vi "649Loops.vi"() -> ()   [LabVIEW 2023]
uses:
  <vilib>/numeric/Random Number (Range) U64.vi
  <vilib>/numeric/sub_Random U32.vi
  <vilib>/Utility/file.llb/Write Delimited Spreadsheet (string).vi
panel:
  in  "Append to file?":bool
  in  "file path (dialog if empty)":path
  out "?":u64[](array[numeric])
  out "?":u64[][](array[numeric])
  in  "?":bool
  # "6@49"
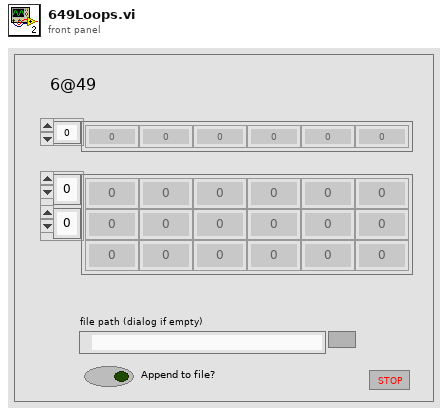
[diagram p1: front panel]
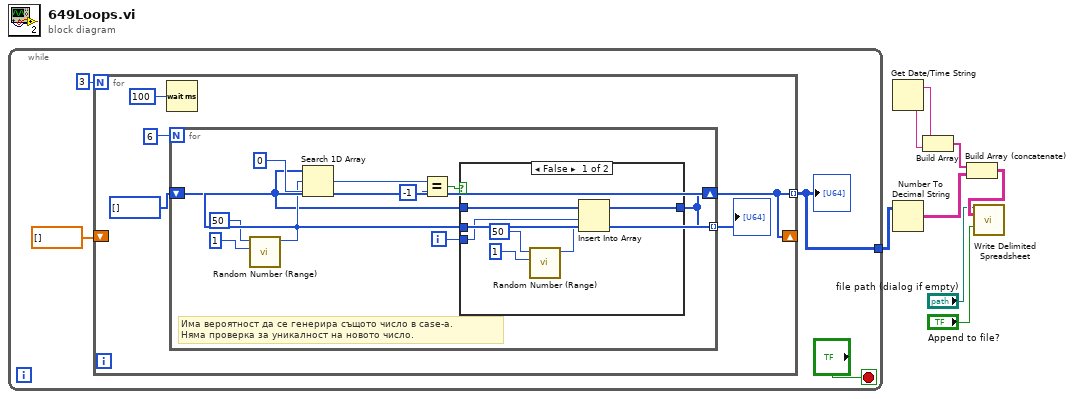
[diagram p0: block diagram]
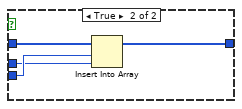
[diagram p2: hidden frame]
diagram:
  n1 = while {
    tunnel: [w9] -> w8
    stop <- "?" stop-if-true
    n2 = for {
      N: 3 -> [_]
      shift-right: [w15] -> _
      shift-left: dbl[] [] ("Array 2") -> [_]
      tunnel: [w15] -> w9 mode=indexing
      n3 = Wait (ms)(milliseconds to wait=u32 100) -> ()  [unwired: 1 out]
      n4 = for {
        N: 6 -> [_]
        tunnel: [w18] -> _ mode=indexing
        shift-right: [w18] -> w15
        shift-left: u64[] [] -> [w17]
        i -> [w20]
        # "Има вероятност да се генерира същото число в case-a.\nНяма проверка за уникалност на новото число."
        n5 = call-poly <vilib>:"Random Number (Range).vi"("lower bound (0)"=u64 1, "upper bound (100)"=u64 50) -> ("number"=w19:u64)  [unwired: 9 in]
        n6 = Search 1D Array(1D array=w17, element=w19, start index (0)=0) -> (index of element=w23:i32)
        n7 = Equal?(x=w23, y=-1) -> (x = y?=w21:bool)
        n8 = case shown="False" w21 {
          tunnel: w17 -> [w28 w36]
          tunnel: w20 -> [w29 w35]
          tunnel: w19 -> [_ w34]
          tunnel: [w27 w33] -> w18
          frame False {
            n9 = call-poly <vilib>:"Random Number (Range).vi"("lower bound (0)"=u64 1, "upper bound (100)"=u64 50) -> ("number"=w30:u64)  [unwired: 9 in]
            n10 = Insert Into Array "Insert Into Array"(array=w28, index=w29, new element=w30) -> (w27:u64[])
          }
          frame True {
            n11 = Insert Into Array "Insert Into Array"(array=w36, index=w35, new element=w34) -> (w33:u64[])
          }
        }
      }
      "?" <- w15
    }
    "?" <- w9
  }
  n12 = Get Date/Time String() -> (date string=w7:string, time string=w6:string)  [unwired: 3 in]
  n13 = Number To Decimal String(number=w8) -> (decimal integer string=w5:string[][])  [unwired: 1 in]
  n14 = Build Array(w7, w6) -> (w4:string[])
  n15 = Build Array (concatenate)(w4, w5) -> (w3:string[][])
  n16 = call-poly <vilib>:"Write Delimited Spreadsheet.vi"("file path (dialog if empty)"="file path (dialog if empty)", "2D data"=w3, "append to file? (new file:F)"="Append to file?") -> ()  [unwired: 11 in, 2 out]
